vi "Open Accelerometer.vi"(4 "ACK Poll Timeout":u16=500, 6 "Clock Rate in kHz":u16=200, 8 "error in (no error)":errorcluster, 10 "I2C address":u16=104 format="%x", 11 "Device":T2="USB0::0x3923::0x7166::01879089::RAW") -> (0 "error out":errorcluster, 3 "Accelerometer":T1)   [LabVIEW 2012]
doc: "Use this template to build a VI to use as a subVI."
uses:
  <vilib>/ni845x/ni845x.llb/ni845xControl.ctl
  Accelerometer.ctl
  <vilib>/ni845x/ni845x.llb/ni845xI2cConfiguration.ctl
  <resource>/objmgr/NI845x.rc
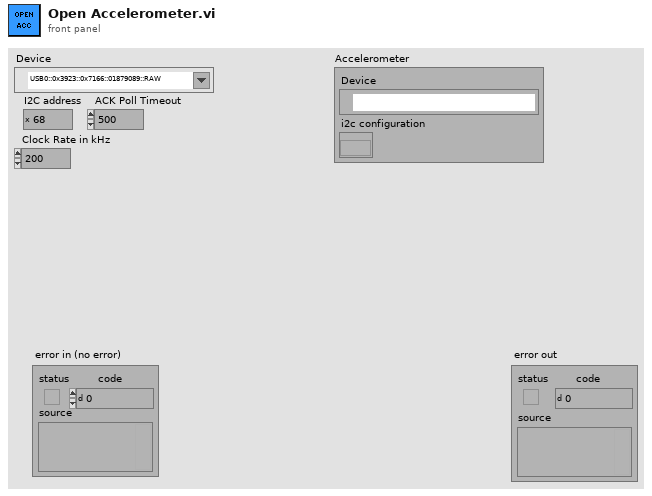
[diagram p1: front panel]
types:
  T1 = typedef "Accelerometer.ctl" = cluster{"Device":T2, "i2c configuration":T3}
  T2 = typedef "ni845xControl.ctl" = refnum<k21>
  T3 = typedef "ni845xI2cConfiguration.ctl" = refnum<k20>
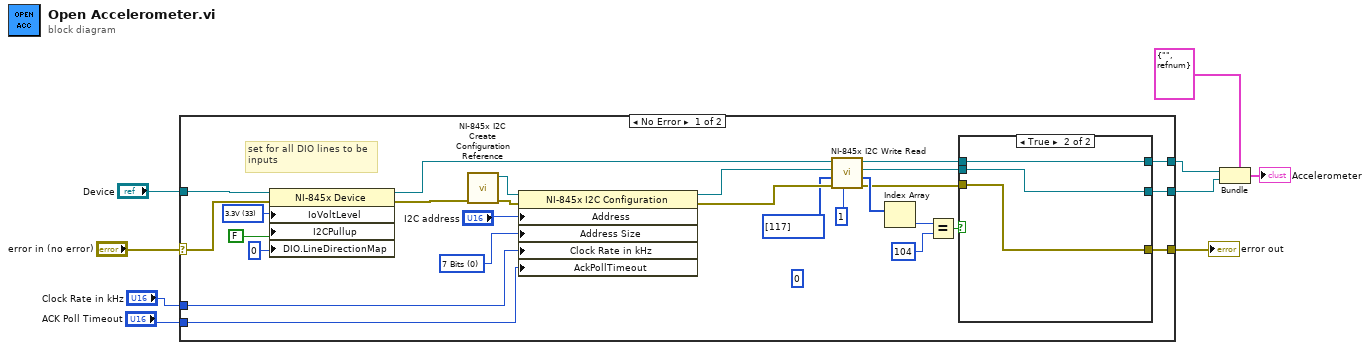
[diagram p0: block diagram]
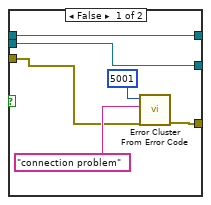
[diagram p2: hidden frame]
diagram:
  n1 = case shown="No Error" "error in (no error)" {
    selector: "error in (no error)" -> [w33 w47]
    tunnel: [w13 w47] -> w8
    tunnel: "Device" -> [w34 w46]
    tunnel: [w15 _] -> w5
    tunnel: [w17 w46] -> w6
    tunnel: "Clock Rate in kHz" -> [w11 _]
    tunnel: "ACK Poll Timeout" -> [w10 _]
    frame No Error {
      (unwired) u8 0
      w30 = 0 items=["7 Bits", "10 Bits"] ("Address Size")
      w35 = 33 items=["3.3V"=33, "2.5V"=25, "1.8V"=18, "1.5V"=15, "1.2V"=12] ("I/O Voltage Level")
      # "set for all DIO lines to be\ninputs"
      n2 = property on="Property Node" class="NI-845x Device"(reference=w34, error in=w33, "IoVoltLevel"=w35, "I2CPullup"=FALSE ("I²C Pullup Enable"), "DIO.LineDirectionMap"=u8 0 ("DIO:Line Direction Map")) -> (reference out=w26:T2, error out=w29:errorcluster)
      n3 = call <vilib>:"NI-845x I2C Create Configuration Reference.vi"("error in (no error)"=w29) -> ("error out"=w31:errorcluster, "i2c configuration"=w32:T3)  [unwired: 9 out]
      n4 = property class="NI-845x I2C Configuration"(reference=w32, error in=w31, "Address"="I2C address", "Address Size"=w30, "Clock Rate in kHz"=w11, "AckPollTimeout"=w10) -> (reference out=w12:T3, error out=w25:errorcluster)
      n5 = call <vilib>:"NI-845x I2C Write Read.vi"("num bytes to read"=u32 1, "error in (no error)"=w25, "write data"=i32[] [117], "i2c configuration in"=w12, "device reference in"=w26) -> ("error out"=w14:errorcluster, "read data"=w22:u8[], "i2c configuration out"=w16:T3, "device reference out"=w18:T2)  [unwired: 3 in]
      n6 = Index Array(array=w22) -> (element=w21:u8)  [unwired: 1 in]
      n7 = Equal?(x=w21, y=104) -> (x = y?=w19:bool)
      n8 = case shown="True" w19 {
        tunnel: w18 -> [w40 w45]
        tunnel: [w40 w45] -> w17
        tunnel: w16 -> [w37 w44]
        tunnel: [w37 w44] -> w15
        tunnel: w14 -> [w39 w43]
        tunnel: [w38 w43] -> w13
        frame False {
          n9 = call <vilib>:"Error Cluster From Error Code.vi"("error in (no error)"=w39, "error message (\"\")"="connection problem" ("error message (\"\")"), "error code (0)"=5001) -> ("error out"=w38:errorcluster)  [unwired: 6 in]
        }
        frame True {
        }
      }
    }
    frame Error {
    }
  }
  "error out" <- w8
  n10 = Bundle(cluster=T1 {"Device"="", "i2c configuration"=refnum} ("Accelerometer"), "Device"=w6, "i2c configuration"=w5) -> (→"Accelerometer":T1)
